vi "Decode MC Packet.vi"(10 "Array":u8[](array[numeric])) -> (2 "xml string":string)   [LabVIEW 2014]
uses:
  CAN/MC/MC Telemetry.ctl
  CAN/MC/MC Temp 1.ctl
  CAN/MC/MC Temp 2.ctl
  CAN/MC/MC Temp 3.ctl
  CAN/MC/MC Current.ctl
  CAN/MC/MC Voltage.ctl
  CAN/MC/MC State.ctl
  CAN/Inverter States.ctl
  CAN/Inverter Run Modes.ctl
  CAN/VSM States.ctl
  CAN/MC/MC Torque.ctl
  CAN/MC/MC Position.ctl
  CAN/MC/MC Faults.ctl
  CAN/MC/MC Flux.ctl
  CAN/MC/MC Internal Voltages.ctl
  CAN/MC/MC Mod Index and Flux Weakening.ctl
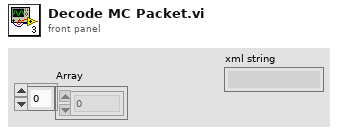
[diagram p1: front panel]
types:
  T1 = typedef "MC Telemetry.ctl" = cluster{"MC Temp 1":T2, "MC Temp 2":T3, "MC Temp 3":T4, "MC Current":T5, "MC Voltage":T6, "MC State":T7, "MC Torque":T11, "MC Position":T12, "MC Faults":T13, "MC Flux":T14, "MC Internal Voltages":T15, "Mod Index & Flux Weakening":T16}
  T2 = typedef "MC Temp 1.ctl" = cluster{"TMCModuleA":dbl, "TMCModuleB":dbl, "TMCModuleC":dbl, "TMCGateDriver":dbl}
  T3 = typedef "MC Temp 2.ctl" = cluster{"TMCControlBoard":dbl, "TMCRTD1":dbl, "TMCRTD2":dbl, "TMCRTD3":dbl}
  T4 = typedef "MC Temp 3.ctl" = cluster{"TMCRTD4":dbl, "TMCRTD5":dbl, "TMotor":dbl, "MTorqueShudder":dbl}
  T5 = typedef "MC Current.ctl" = cluster{"IMCPhaseA":dbl, "IMCPhaseB":dbl, "IMCPhaseC":dbl, "IMCBatteryCalc":dbl}
  T6 = typedef "MC Voltage.ctl" = cluster{"VMCPhaseAB":dbl, "VMCPhaseBC":dbl, "VMCOutput":dbl, "VMCBattery":dbl}
  T7 = typedef "MC State.ctl" = cluster{"eMCInverterState":T8, "eMCInverterRunMode":T9, "eMCInverterCommandMode":enum16{"CAN Mode", "VSM Mode"}, "bMCInverterEnable":bool, "bMCInverterEnableLockout":bool, "bMCDirectionForward":bool, "eMCVSMState":T10, "bMCRelay1":bool, "bMCRelay2":bool, "bMCRelay3":bool, "bMCRelay4":bool}
  T8 = typedef "Inverter States.ctl" = enum16{"Power On", "Stop", "Open Loop", "Closed Loop", "Wait", "Internal", "Idle Run", "Idle Stop", ""}
  T9 = typedef "Inverter Run Modes.ctl" = enum16{"Torque Mode", "Speed Mode"}
  T10 = typedef "VSM States.ctl" = enum16{"VSM Start", "Pre-Charge Init", "Pre-Charge Active", "Pre-Charge Complete", "VSM Wait", "VSM Ready", "Motor Running", "Blink Fault Code", "Shutdown in Process", "Recycle Power"}
  T11 = typedef "MC Torque.ctl" = cluster{"MMCRequested":dbl, "MMCFeedback":dbl, "tMCElapsed":u32}
  T12 = typedef "MC Position.ctl" = cluster{"aMotor":dbl, "nMotor":dbl, "fMCOutput":dbl, "aDeltaResolverFilt":dbl}
  T13 = typedef "MC Faults.ctl" = cluster{"MC Fault":cluster{"Over-Speed":bool, "Over-Current":bool, "Over-Voltage":bool, "Inverter Over-Temp":bool, "Direction Command":bool, "Inverter Response Time-Out":bool, "Desat Fault":bool, "Hardware Over-Current":bool, "Under-Voltage":bool, "CAN Command Message Lost":bool, "Motor Over-Temp":bool, "Module A Over-Temp":bool, "Module B Over-Temp":bool, "Module C Over-Temp":bool, "PCB Over-Temp":bool, "Gate Driver 1 Over-Temp":bool, "Gate Driver 2 Over-Temp":bool, "Gate Drive 3 Over-Temp":bool, "Current Sensor Fault":bool, "Resolver Not Connected":bool}, "MC Post":u32, "MC RUN":u32}
  T14 = typedef "MC Flux.ctl" = cluster{"IMCFluxCommand":dbl, "IMCFluxFeedback":dbl, "IMC_Id":dbl, "IMC_Iq":dbl}
  T15 = typedef "MC Internal Voltages.ctl" = cluster{"VMCRef1_5":dbl, "VMCRef2_5":dbl, "VMCRef5":dbl, "VMCRef12":dbl}
  T16 = typedef "MC Mod Index and Flux Weakening.ctl" = cluster{"NMCModulationIndex":dbl, "IMCFluxWeakeningOutput":dbl, "IMCIdCommand":dbl, "IMCIqCommand":dbl}
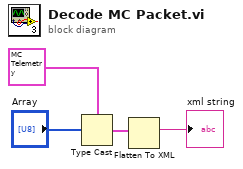
[diagram p0: block diagram]
diagram:
  n1 = Type Cast(type=T1 {"MC Temp 1"={"TMCModuleA"=0.0, "TMCModuleB"=0.0, "TMCModuleC"=0.0, "TMCGateDriver"=0.0}, "MC Temp 2"={"TMCControlBoard"=0.0, "TMCRTD1"=0.0, "TMCRTD2"=0.0, "TMCRTD3"=0.0}, "MC Temp 3"={"TMCRTD4"=0.0, "TMCRTD5"=0.0, "TMotor"=0.0, "MTorqueShudder"=0.0}, "MC Current"={"IMCPhaseA"=0.0, "IMCPhaseB"=0.0, "IMCPhaseC"=0.0, "IMCBatteryCalc"=0.0}, "MC Voltage"={"VMCPhaseAB"=0.0, "VMCPhaseBC"=0.0, "VMCOutput"=0.0, "VMCBattery"=0.0}, "MC State"={"eMCInverterState"=enum."Power On", "eMCInverterRunMode"=enum."Torque Mode", "eMCInverterCommandMode"=enum."CAN Mode", "bMCInverterEnable"=FALSE, "bMCInverterEnableLockout"=FALSE, "bMCDirectionForward"=FALSE, "eMCVSMState"=enum."VSM Start", "bMCRelay1"=FALSE, "bMCRelay2"=FALSE, "bMCRelay3"=FALSE, "bMCRelay4"=FALSE}, "MC Torque"={"MMCRequested"=0.0, "MMCFeedback"=0.0, "tMCElapsed"=0}, "MC Position"={"aMotor"=0.0, "nMotor"=0.0, "fMCOutput"=0.0, "aDeltaResolverFilt"=0.0}, "MC Faults"={"MC Fault"={"Over-Speed"=FALSE, "Over-Current"=FALSE, "Over-Voltage"=FALSE, "Inverter Over-Temp"=FALSE, "Direction Command"=FALSE, "Inverter Response Time-Out"=FALSE, "Desat Fault"=FALSE, "Hardware Over-Current"=FALSE, "Under-Voltage"=FALSE, "CAN Command Message Lost"=FALSE, "Motor Over-Temp"=FALSE, "Module A Over-Temp"=FALSE, "Module B Over-Temp"=FALSE, "Module C Over-Temp"=FALSE, "PCB Over-Temp"=FALSE, "Gate Driver 1 Over-Temp"=FALSE, "Gate Driver 2 Over-Temp"=FALSE, "Gate Drive 3 Over-Temp"=FALSE, "Current Sensor Fault"=FALSE, "Resolver Not Connected"=FALSE}, "MC Post"=0, "MC RUN"=0}, "MC Flux"={"IMCFluxCommand"=0.0, "IMCFluxFeedback"=0.0, "IMC_Id"=0.0, "IMC_Iq"=0.0}, "MC Internal Voltages"={"VMCRef1_5"=0.0, "VMCRef2_5"=0.0, "VMCRef5"=0.0, "VMCRef12"=0.0}, "Mod Index & Flux Weakening"={"NMCModulationIndex"=0.0, "IMCFluxWeakeningOutput"=0.0, "IMCIdCommand"=0.0, "IMCIqCommand"=0.0}} ("MC Telemetry"), x="Array") -> (*(type *) &x=w3:T1)
  n2 = Flatten To XML(anything=w3) -> (xml string=→"xml string":string)
